vi "getXMLTestCases (Extended).vi"(9 "indent level":i32, 10 "testcases":T1[](array[typedef]), 11 "Test Report in":refnum<class "Test Report.lvclass">) -> (2 "XML testcases":string[](array[string]), 3 "Test Report":refnum<class "Test Report.lvclass">)   [LabVIEW 2013, in "Caraya.lvlib" / "Test Report.JUnit.lvclass"]
uses:
  Test Report.JUnit.lvclass
  extended -- cluster.ctl
  Test Report/Test Report.lvclass
  Test Report/Test Report.lvclass/Test Report.ctl
  MsgSerializer/MsgSerializer.lvclass/MsgSerializer.ctl
  MsgSerializer/MsgSerializer.lvclass
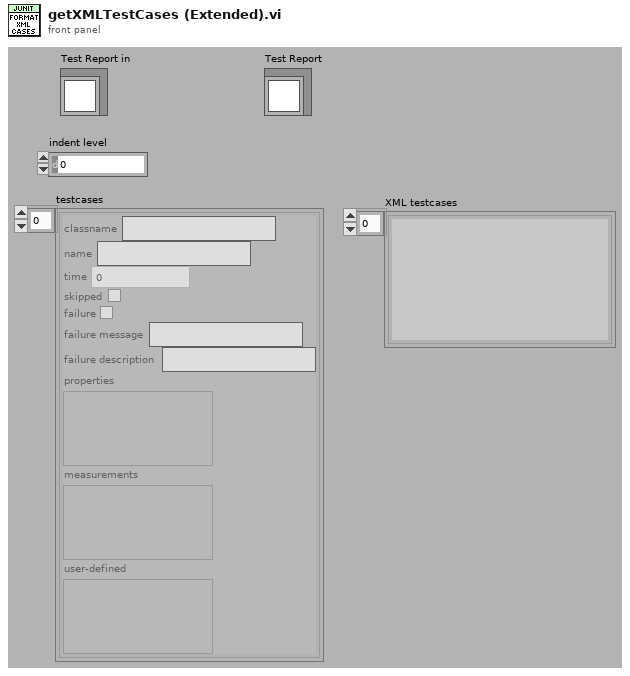
[diagram p1: front panel]
types:
  T1 = typedef "Caraya.lvlib/Test Report.JUnit.lvclass/extended -- cluster.ctl" = cluster{"classname":string, "name":string, "time":dbl, "skipped":bool, "failure":bool, "failure message":string, "failure description":string, "properties":variant, "measurements":variant, "user-defined":variant}
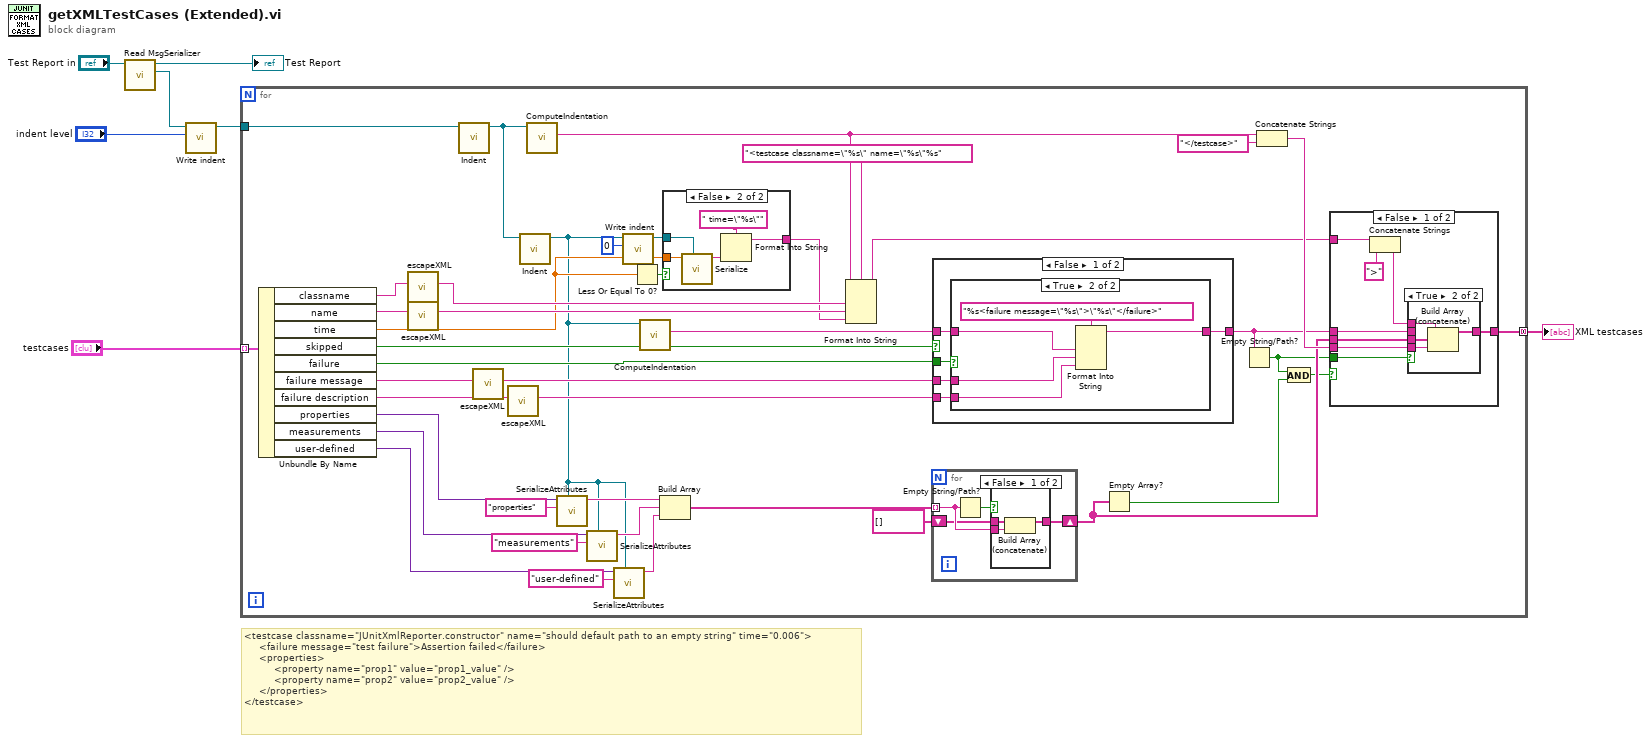
[diagram p0: block diagram]
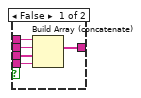
[diagram p4: hidden frame]
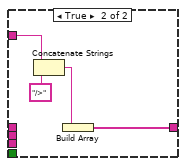
[diagram p5: hidden frame]
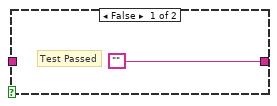
[diagram p6: hidden frame]
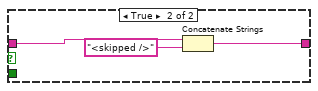
[diagram p7: hidden frame]
diagram:
  # "<testcase classname=\"JUnitXmlReporter.constructor\" name=\"should default path to an empty string\" time=\"0.006\">\n     <failure message=\"test failure\">Assertion failed</failure>\n     <properties>\n          <property name=\"prop1\" value=\"prop1_value\" />\n          <property name=\"prop2\" value=\"prop2_value\" />\n     </properties>\n</testcase>"
  n1 = call "Read MsgSerializer.vi"("Test Report in"="Test Report in") -> ("MsgSerializer"=w3:refnum<class "MsgSerializer.lvclass">, "Test Report out"=→"Test Report":refnum<class "Test Report.lvclass">)  [unwired: 9 in]
  n2 = call "Write indent.vi"("indent"="indent level", "MsgSerializer in"=w3) -> ("MsgSerializer out"=w2:refnum<class "MsgSerializer.lvclass">)  [unwired: 9 in]
  n3 = for {
    tunnel: "testcases" -> [w49] mode=indexing
    tunnel: [w18] -> w6 mode=concatenating
    tunnel: w2 -> [w27]
    n4 = Unbundle By Name(w49) -> ("classname"=w46:string, "name"=w44:string, "time"=w12:dbl, "skipped"=w48:bool, "failure"=w47:bool, "failure message"=w42:string, "failure description"=w40:string, "properties"=w34:variant, "measurements"=w36:variant, "user-defined"=w31:variant)
    n5 = call "escapeXML.vi"("Input String"=w46) -> ("XML-escaped String"=w45:string)  [unwired: 10 in]
    n6 = call "escapeXML.vi"("Input String"=w44) -> ("XML-escaped String"=w43:string)  [unwired: 10 in]
    n7 = call "Indent.vi"("MsgSerializer in"=w27) -> ("MsgSerializer out"=w26:refnum<class "MsgSerializer.lvclass">)  [unwired: 10 in]
    n8 = call "escapeXML.vi"("Input String"=w42) -> ("XML-escaped String"=w41:string)  [unwired: 10 in]
    n9 = call "escapeXML.vi"("Input String"=w40) -> ("XML-escaped String"=w39:string)  [unwired: 10 in]
    n10 = call "Indent.vi"("MsgSerializer in"=w26) -> ("MsgSerializer out"=w8:refnum<class "MsgSerializer.lvclass">)  [unwired: 10 in]
    n11 = call "ComputeIndentation.vi"("MsgSerializer in"=w26) -> ("indentation"=w10:string)  [unwired: 10 in]
    n12 = call "SerializeAttributes.vi"("MsgSerializer"=w8, "attribute name"="properties", "variant attribute"=w34) -> ("Serialized Message"=w24:string)  [unwired: 8 in]
    n13 = call "SerializeAttributes.vi"("MsgSerializer"=w8, "attribute name"="measurements", "variant attribute"=w36) -> ("Serialized Message"=w23:string)  [unwired: 8 in]
    n14 = call "SerializeAttributes.vi"("MsgSerializer"=w8, "attribute name"="user-defined", "variant attribute"=w31) -> ("Serialized Message"=w22:string)  [unwired: 8 in]
    n15 = call "Write indent.vi"("indent"=0, "MsgSerializer in"=w8) -> ("MsgSerializer out"=w11:refnum<class "MsgSerializer.lvclass">)  [unwired: 9 in]
    n16 = Less Or Equal To 0?(x=w12) -> (x <= 0?=w29:bool)
    n17 = call "ComputeIndentation.vi"("MsgSerializer in"=w8) -> ("indentation"=w25:string)  [unwired: 10 in]
    n18 = Build Array(w24, w23, w22) -> (w20:string[])
    n19 = case shown="False" w29 {
      tunnel: [_ w61] -> w30
      tunnel: w12 -> [_ w60]
      tunnel: w11 -> [_ w58]
      frame True {
      }
      frame False {
        n20 = call-dynamic "Serialize.vi"("MsgSerializer"=w58, "Value"=w60) -> ("Serialized Message"=w59:string)  [unwired: 8 in, 1 out]
        n21 = Format Into String(format string=" time=\"%s\"", w59) -> (resulting string=w61:string)  [unwired: 2 in, 1 out]
      }
    }
    n22 = Format Into String(format string="<testcase classname=\"%s\" name=\"%s\"%s", initial string=w10, w45, w43, w30) -> (resulting string=w13:string)  [unwired: 1 in, 1 out]
    n23 = for {
      shift-right: [w51] -> w19
      shift-left: string[] [] -> [w52]
      tunnel: w20 -> [w53] mode=indexing
      n24 = Empty String/Path?(string/path=w53) -> (empty?=w50:bool)
      n25 = case shown="False" w50 {
        tunnel: [w56 w57] -> w51
        tunnel: w52 -> [w55 w57]
        tunnel: w53 -> [w54 _]
        frame False {
          n26 = Build Array (concatenate)(w55, w54) -> (w56:string[])
        }
        frame True {
        }
      }
    }
    n27 = case shown="False" w48 {
      tunnel: w47 -> [w88 _]
      tunnel: w41 -> [w87 _]
      tunnel: w39 -> [w86 _]
      tunnel: w25 -> [w85 w96]
      tunnel: [w84 w95] -> w14
      frame False {
        n28 = case shown="True" w88 {
          tunnel: w87 -> [_ w93]
          tunnel: w86 -> [_ w92]
          tunnel: w85 -> [_ w91]
          tunnel: ["" w90] -> w84
          frame False {
            # "Test Passed"
          }
          frame True {
            n29 = Format Into String(format string="%s<failure message=\"%s\">\"%s\"</failure>", w91, w93, w92) -> (resulting string=w90:string)  [unwired: 2 in, 1 out]
          }
        }
      }
      frame True {
        n30 = Concatenate Strings(w96, "<skipped />") -> (w95:string)
      }
    }
    n31 = Empty Array?(array=w19) -> (empty?=w17:bool)
    n32 = Empty String/Path?(string/path=w14) -> (empty?=w15:bool)
    n33 = Concatenate Strings(w10, "</testcase>") -> (w37:string)
    n34 = And(x=w15, y=w17) -> (x .and. y?=w16:bool)
    n35 = case shown="False" w16 {
      tunnel: w13 -> [w69 w81]
      tunnel: [w66 w80] -> w18
      tunnel: w37 -> [w65 _]
      tunnel: w14 -> [w67 _]
      tunnel: w19 -> [w64 _]
      tunnel: w15 -> [w63 _]
      frame False {
        n36 = Concatenate Strings(w69, ">" ("string")) -> (w68:string)
        n37 = case shown="True" w63 {
          tunnel: w68 -> [w75 w77]
          tunnel: w67 -> [w74 _]
          tunnel: [w73 w76] -> w66
          tunnel: w65 -> [w72 w79]
          tunnel: w64 -> [w71 w78]
          frame False {
            n38 = Build Array (concatenate)(w75, w74, w71, w72) -> (w73:string[])
          }
          frame True {
            n39 = Build Array (concatenate)(w77, w78, w79) -> (w76:string[])
          }
        }
      }
      frame True {
        n40 = Concatenate Strings(w81, "/>" ("string")) -> (w83:string)
        n41 = Build Array(w83) -> (w80:string[])
      }
    }
  }
  "XML testcases" <- w6
